vi "LibXML_UnlinkNode.vi"(8 "error in":errorcluster, 11 "node":u32) -> (0 "error out":errorcluster, 3 "node copy out":u32)   [LabVIEW 2019, in "Tools.lvlib" / "LibXML.lvlib"]
doc: "void xmlUnlinkNode (xmlNodePtr cur)\n\nUnlink a node from it's current context, the node is not freed\ncur: the node"
uses:
  LibXML.lvlib
  dll/libxml2.dll
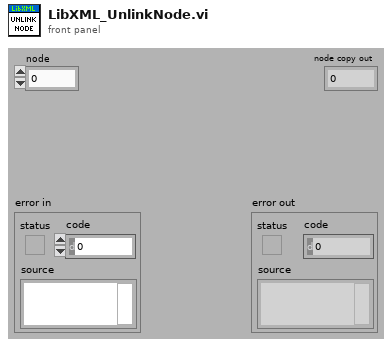
[diagram p1: front panel]
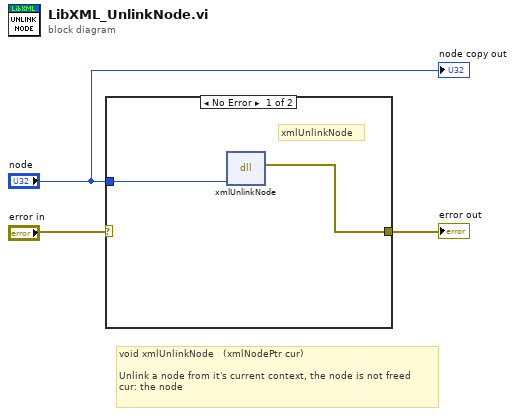
[diagram p0: block diagram]
diagram:
  # "void\txmlUnlinkNode\t\t\t(xmlNodePtr cur)\n\nUnlink a node from it's current context, the node is not freed\ncur:\tthe node"
  n1 = case shown="No Error" "error in" {
    selector: "error in" -> [_ w6]
    tunnel: [w4 w6] -> w2
    tunnel: "node" -> [w5 _]
    frame No Error {
      # "xmlUnlinkNode"
      n2 = dll-call lib="C:/Projects/_Prywatne/MyCIT/Framework/Tools/XML/LibXML/dll/libxml2.dll" fn="xmlUnlinkNode"("node"=w5) -> (error out=w4:errorcluster)  [unwired: 5 in, 1 out]
    }
    frame Error {
    }
  }
  "error out" <- w2
  "node copy out" <- "node"
